vi "To Serial Form.vi"(6 "Serial Version":T1, 10 "Serializer in":refnum<class "Serializer.lvclass">, 11 "cPAS in":refnum<class "cPAS.lvclass">) -> (0 "error out":errorcluster, 2 "Serializer out":refnum<class "Serializer.lvclass">, 3 "cPAS out":refnum<class "cPAS.lvclass">)   [LabVIEW 2012]
uses:
  <userlib>/Serialization/Serializable/Serializable.lvclass
  <userlib>/Serialization/Serializable/Insert Serializable.vi
  <userlib>/Serialization/Serializable/Insert Single Array.vi
  <userlib>/Serialization/Serializable/Insert Boolean Array.vi
  <userlib>/Serialization/Serializable/Insert Single.vi
  <userlib>/Serialization/Serializable/Insert Boolean.vi
  <userlib>/Serialization/Serializer/Serializer.lvclass
  <userlib>/Serialization/Serialization Common/Serial Version.ctl
  <userlib>/Serialization/Serialization Common/Serialization Common.lvlib
  cPAS.lvclass
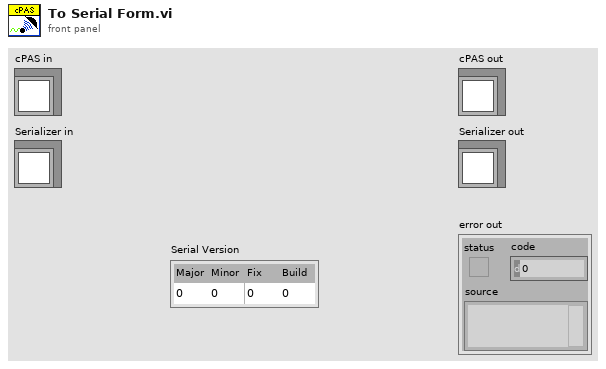
[diagram p1: front panel]
types:
  T1 = typedef "Serialization Common.lvlib/Serial Version.ctl" = cluster{"Major":u16, "Minor":u16, "Fix":u16, "Build":u16}
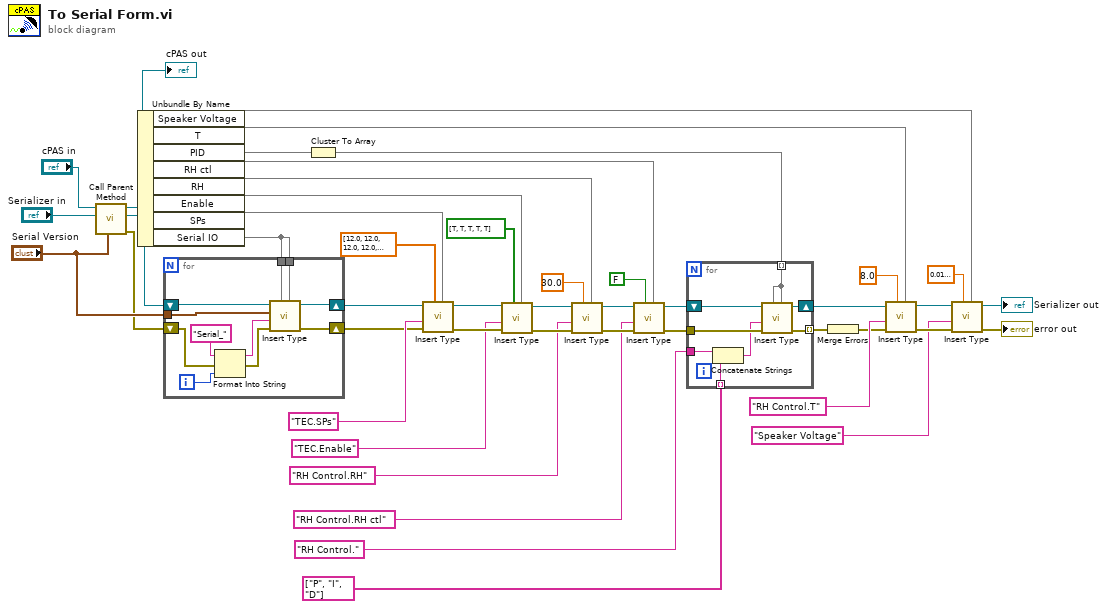
[diagram p0: block diagram]
diagram:
  n1 = call-parent "Call Parent Method"("Serial Version"="Serial Version", "Serializer in"="Serializer in", "PAS in"="cPAS in") -> ("error out"=w40:errorcluster, "Serializer out"=w42:refnum<class "Serializer.lvclass">, "PAS out"=w44:refnum<class "cPAS.lvclass">)  [unwired: 6 in]
  "cPAS out" <- w44
  n2 = Unbundle By Name(w44) -> ("Speaker Voltage"=w3, "T"=w8, "PID"=w16, "RH ctl"=w20, "RH"=w28, "Enable"=w33, "SPs"=w37, "Serial IO"=w43)
  n3 = for {
    tunnel: w43 -> [w57]
    tunnel: w43 -> [w56]
    tunnel: "Serial Version" -> [w54]
    shift-right: [w50] -> w36
    shift-left: w40 -> [w48]
    shift-right: [w49] -> w39
    shift-left: w42 -> [w55]
    i -> [w53]
    n4 = Format Into String(initial string="Serial_", error in=w48, w53) -> (resulting string=w51:string, error out=w47:errorcluster)  [unwired: 1 in]
    n5 = call-poly <userlib>:"Insert Type.vi"("Serializable"=w57, "Default Value"=w56, "error in (no error)"=w47, "Name"=w51, "Serial Version"=w54, "Serializer in"=w55) -> ("error out"=w50:errorcluster, "Serializer out"=w49:refnum<class "Serializer.lvclass">)  [unwired: 4 in]
  }
  n6 = Cluster To Array(cluster=w16) -> (array=w15:void[])
  n7 = call-poly <userlib>:"Insert Type.vi"("Singles"=w37, "Default Value"=sgl[] [12.0, 12.0, 12.0, 12.0, 12.0], "error in (no error)"=w36, "Name"="TEC.SPs", "Serializer in"=w39) -> ("error out"=w34:errorcluster, "Serializer out"=w35:refnum<class "Serializer.lvclass">)  [unwired: 5 in]
  n8 = call-poly <userlib>:"Insert Type.vi"("Booleans"=w33, "Default Value"=bool[] [TRUE, TRUE, TRUE, TRUE, TRUE], "error in (no error)"=w34, "Name"="TEC.Enable", "Serializer in"=w35) -> ("error out"=w26:errorcluster, "Serializer out"=w29:refnum<class "Serializer.lvclass">)  [unwired: 5 in]
  n9 = call-poly <userlib>:"Insert Type.vi"("Double"=w28, "Default Value"=sgl 30.0, "error in (no error)"=w26, "Name"="RH Control.RH", "Serializer in"=w29) -> ("error out"=w24:errorcluster, "Serializer out"=w25:refnum<class "Serializer.lvclass">)  [unwired: 5 in]
  n10 = call-poly <userlib>:"Insert Type.vi"("Boolean"=w20, "Default Value"=FALSE, "error in (no error)"=w24, "Name"="RH Control.RH ctl", "Serializer in"=w25) -> ("error out"=w18:errorcluster, "Serializer out"=w19:refnum<class "Serializer.lvclass">)  [unwired: 5 in]
  n11 = for {
    tunnel: w18 -> [w64]
    shift-right: [w63] -> w12
    shift-left: w19 -> [w65]
    tunnel: string[] ["P", "I", "D"] -> [w61] mode=indexing
    tunnel: w15 -> [w62] mode=indexing
    tunnel: "RH Control." -> [w60]
    tunnel: [w58] -> w13 mode=indexing
    n12 = Concatenate Strings(w60, w61) -> (w59:string)
    n13 = call-poly <userlib>:"Insert Type.vi"("Double"=w62, "Default Value"=w62, "error in (no error)"=w64, "Name"=w59, "Serializer in"=w65) -> ("error out"=w58:errorcluster, "Serializer out"=w63:refnum<class "Serializer.lvclass">)  [unwired: 5 in]
  }
  n14 = Merge Errors(w13) -> (w10:errorcluster)
  n15 = call-poly <userlib>:"Insert Type.vi"("Double"=w8, "Default Value"=sgl 8.0, "error in (no error)"=w10, "Name"="RH Control.T", "Serializer in"=w12) -> ("error out"=w6:errorcluster, "Serializer out"=w7:refnum<class "Serializer.lvclass">)  [unwired: 5 in]
  n16 = call-poly <userlib>:"Insert Type.vi"("Double"=w3, "Default Value"=sgl 0.02, "error in (no error)"=w6, "Name"="Speaker Voltage", "Serializer in"=w7) -> ("error out"=→"error out":errorcluster, "Serializer out"=→"Serializer out":refnum<class "Serializer.lvclass">)  [unwired: 5 in]
